vi "Write Discrete Inputs.vi"(8 "error in (no error)":errorcluster, 9 "input values":bool[](array[boolean]), 10 "starting address":u16, 11 "Standard Data Model in":refnum<class "Standard Data Model.lvclass">) -> (0 "error out":errorcluster, 3 "Standard Data Model out":refnum<class "Standard Data Model.lvclass">)   [LabVIEW 2013, in "Modbus Library - Advance.lvlib" / "Standard Data Model.lvclass"]
doc: "Writes the values of multiple discrete input values in series, starting at address M."
uses:
  Standard Data Model.lvclass
  Standard Data Model.lvclass/Standard Data Model.ctl
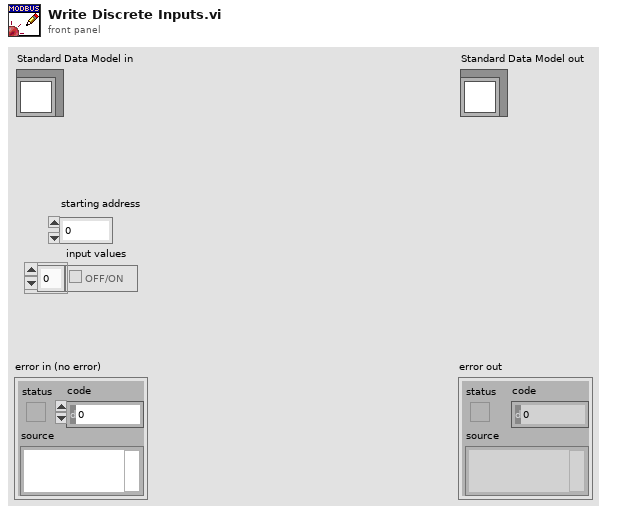
[diagram p1: front panel]
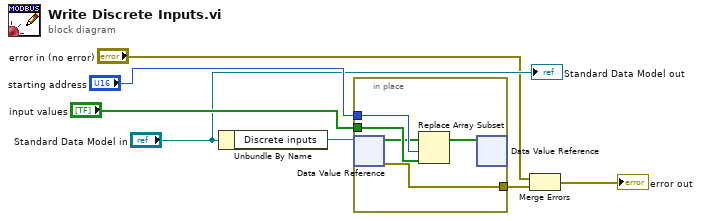
[diagram p0: block diagram]
diagram:
  n1 = Unbundle By Name("Standard Data Model in") -> ("Discrete inputs"=w5:refnum<data-value>)
  n2 = in-place {
    in-place-border: "starting address" -> [w12]
    in-place-border: "input values" -> [w11]
    in-place-border: [w8] -> w1
    n3 = in-place-dvr #1(w5) -> (w10:bool[], w8:errorcluster)
    n4 = Replace Array Subset(array=w10, new element=w11, index=w12) -> (w9:bool[])
    n5 = in-place-dvr #1(w9) -> ()  [unwired: 2 out]
  }
  n6 = Merge Errors("error in (no error)", w1) -> (→"error out":errorcluster)
  "Standard Data Model out" <- "Standard Data Model in"
